vi "extract From Input Packet msg CNT.vi"(11 "instance":i32) -> (3 "function return":u32)   [LabVIEW 2025, in "SADI_FW3.lvlib"]
doc: "SADI_API_Wrapper uint32_t extractFromInputPacket_msgCNT(int instance);"
uses:
  SADI_FW3.lvlib
  SADI_FW3.dll
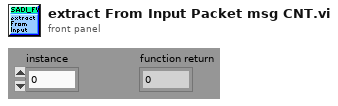
[diagram p1: front panel]
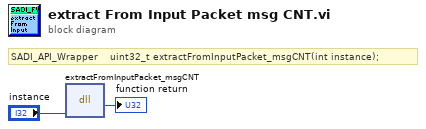
[diagram p0: block diagram]
diagram:
  # "SADI_API_Wrapper    uint32_t extractFromInputPacket_msgCNT(int instance);"
  n1 = dll-call lib="C:/Users/noaht/School/Fall 2025/Controls Lab/Lab 3/EML4314c_FA25_framework_0/LVLib/SADI_FW3.*" fn="extractFromInputPacket_msgCNT"("instance"="instance") -> ("return type"=→"function return":u32)  [unwired: 4 in, 2 out]
